vi "周期设置.vi"(11 "定时控制参数输入":T1) -> (3 "定时控制参数输出":T1)   [LabVIEW 2016, in "质控单元.lvlib"]
uses:
  <vilib>/Utility/miscctls.llb/LVPointTypeDef.ctl
panel:
  in  "采配水启用":bool
  in  "模块选择":T2
  in  "确定":bool
  in  "取消":bool
  in  "定时功能启用":bool
  out "选项卡控件":enum32{"定点启动", "间隔启动"}(tab)
  in  "24H周期设置":bool[](xcontrol)
  in  "已经启动次数":dbl
  in  "设定启动次数":dbl
  in  "定时间隔":dbl
  in  "周期设置类型":enum16{"定点启动", "间隔启动"}(ring)
  # "仪器测试类型："
  # "周期设置类型："
  # "请输入定时启动间隔"
  # "min"
  # "次"
  # "次"
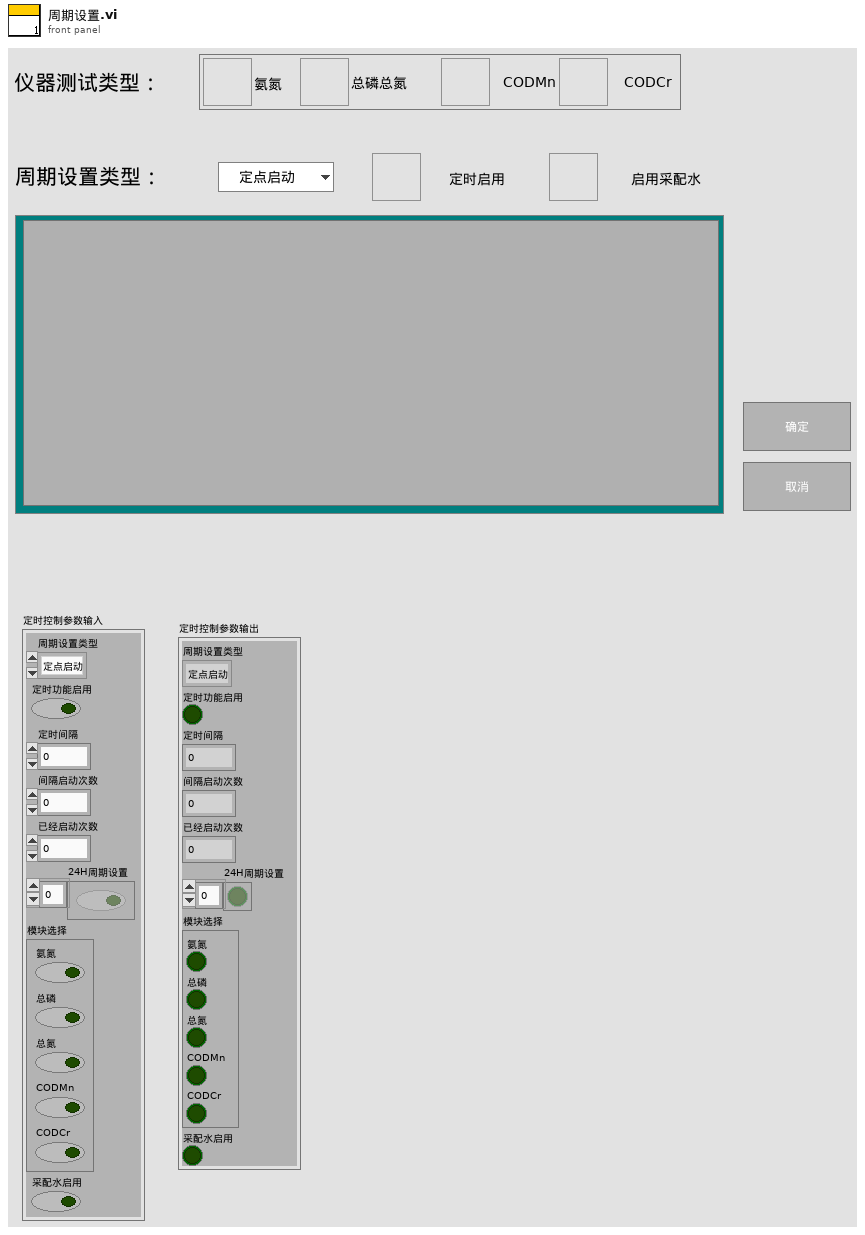
[diagram p1: front panel]
types:
  T1 = cluster{"周期设置类型":enum16{"定点启动", "间隔启动"}, "定时功能启用":bool, "定时间隔":dbl, "间隔启动次数":dbl, "已经启动次数":dbl, "24H周期设置":bool[], "模块选择":cluster{"氨氮":bool, "总磷":bool, "总氮":bool, "CODMn":bool, "CODCr":bool}, "采配水启用":bool}
  T2 = cluster{"氨氮":bool, "总磷":bool, "总氮":bool, "CODMn":bool, "CODCr":bool}
  T3 = typedef "LVPointTypeDef.ctl" = cluster{"Horizontal":i16, "Vertical":i16}
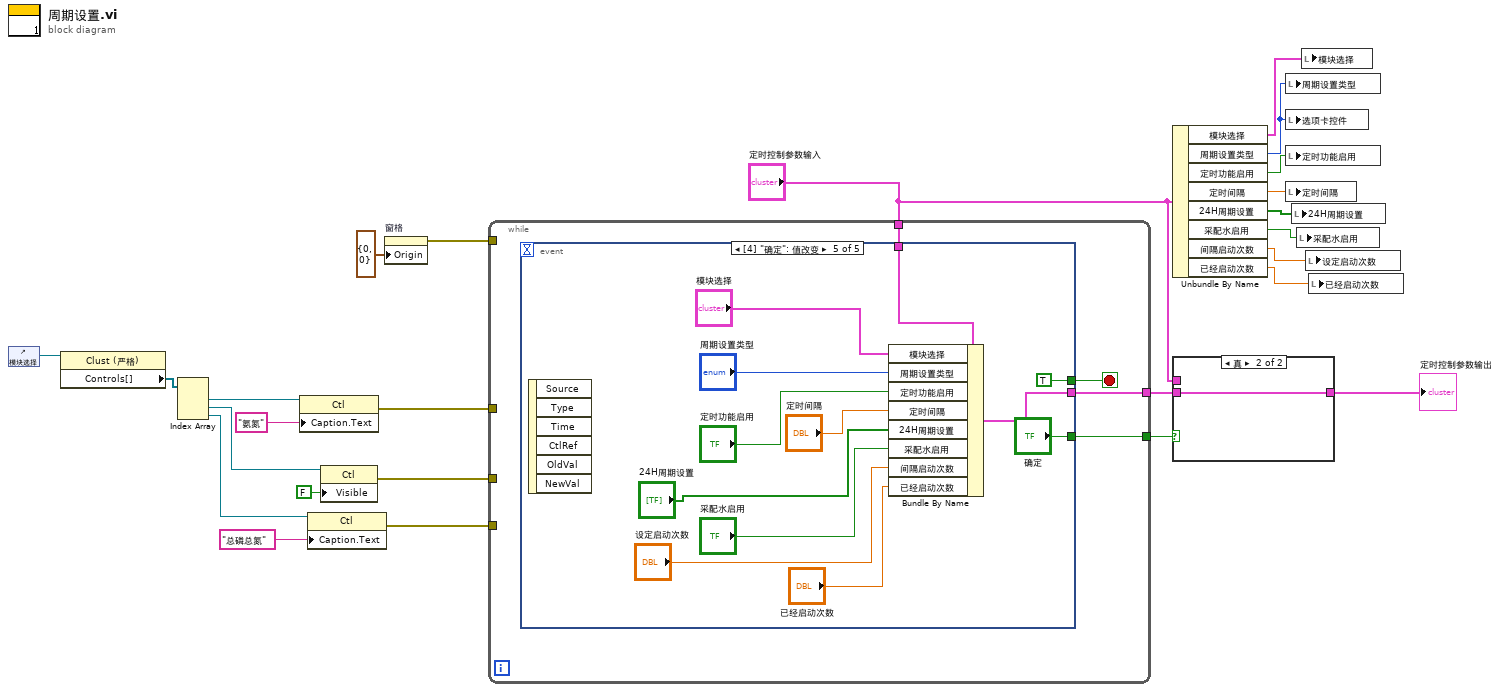
[diagram p0: block diagram]
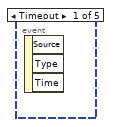
[diagram p3: hidden frame]
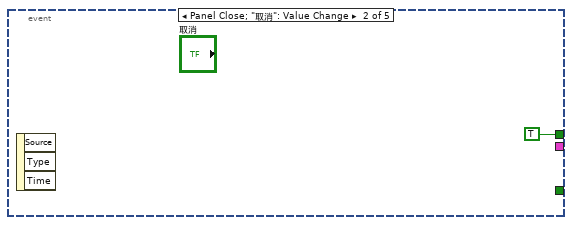
[diagram p4: hidden frame]
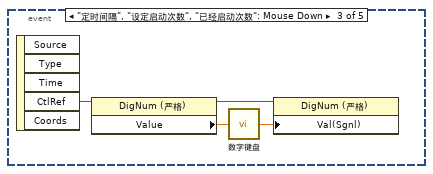
[diagram p5: hidden frame]
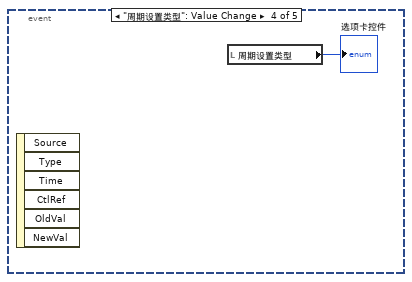
[diagram p6: hidden frame]
diagram:
  n1 = control-ref of="模块选择"() -> (w11:refnum<vi>)
  n2 = property class="Clust (严格)"(reference=w11) -> ("Controls[]"=w9:refnum<vi>[])  [unwired: 1 in, 2 out]
  n3 = Index Array(array=w9) -> (element #1=w10:refnum<vi>, element #2=w7:refnum<vi>, element #3=w2:refnum<vi>)  [unwired: 3 in]
  n4 = property class="Ctl"(reference=w10, "Caption.Text"="氨氮" ("标题.文本")) -> (error out=w5:errorcluster)  [unwired: 1 in, 1 out]
  n5 = property class="Ctl"(reference=w2, "Caption.Text"="总磷总氮" ("标题.文本")) -> (error out=w1:errorcluster)  [unwired: 1 in, 1 out]
  n6 = property class="Ctl"(reference=w7, "Visible"=FALSE ("可见")) -> (error out=w4:errorcluster)  [unwired: 1 in, 1 out]
  n7 = property on="窗格" class="Pane"("Origin"=T3 {"Horizontal"=0, "Vertical"=0} ("原点")) -> (error out=w14:errorcluster)  [unwired: 2 in, 1 out]
  n8 = while {
    tunnel: [w28] -> w20
    tunnel: [w27] -> w21
    tunnel: "定时控制参数输入" -> [w26]
    tunnel: w14 -> [_]
    tunnel: w5 -> [_]
    tunnel: w4 -> [_]
    tunnel: w1 -> [_]
    stop <- w29 stop-if-true
    n9 = event shown="[4] \"确定\": 值改变" {
      selector: _ -> [_ _ _ _ _]
      dyn-events: _ -> [_ _ _ _ _]
      timeout: _ -> [_ _ _ _ _]
      tunnel: [_ TRUE _ _ TRUE] -> w29
      tunnel: [_ _ _ _ w44] -> w28
      tunnel: [_ _ _ _ "确定"] -> w27
      tunnel: w26 -> [_ _ _ _ w39]
      event Timeout {
        n10 = event-data() -> ()  [unwired: 1 in, 3 out]
      }
      event Panel Close; "取消": Value Change {
        n11 = event-data() -> ()  [unwired: 1 in, 3 out]
      }
      event "定时间隔", "设定启动次数", "已经启动次数": Mouse Down {
        n12 = event-data() -> ("CtlRef"=w34:refnum<vi>)  [unwired: 1 in, 4 out]
        n13 = property class="DigNum (严格)"(reference=w34) -> (reference out=w31:refnum<vi>, "Value"=w33:dbl)  [unwired: 1 in, 1 out]
        n14 = call "数字键盘.vi"("OldNumber"=w33) -> ("NewNumber"=w32:sgl)
        n15 = property class="DigNum (严格)"(reference=w31, "Val(Sgnl)"=w32) -> ()  [unwired: 1 in, 2 out]
      }
      event "周期设置类型": Value Change {
        n16 = event-data() -> ()  [unwired: 1 in, 6 out]
        n17 = local read "周期设置类型"() -> (→"选项卡控件":enum16{"定点启动", "间隔启动"})
      }
      event "确定": Value Change {
        n18 = event-data() -> ()  [unwired: 1 in, 6 out]
        n19 = Bundle By Name(cluster=w39, "模块选择"="模块选择", "周期设置类型"="周期设置类型", "定时功能启用"="定时功能启用", "定时间隔"="定时间隔", "24H周期设置"="24H周期设置", "采配水启用"="采配水启用", "间隔启动次数"="设定启动次数", "已经启动次数"="已经启动次数") -> (w44:T1)
      }
    }
  }
  n20 = Unbundle By Name("定时控制参数输入") -> ("模块选择"=w19:T2, "周期设置类型"=w22:enum16{"定点启动", "间隔启动"}, "定时功能启用"=w25:bool, "定时间隔"=w24:dbl, "24H周期设置"=w23:bool[], "采配水启用"=w17:bool, "间隔启动次数"=w13:dbl, "已经启动次数"=w12:dbl)
  n21 = case shown="真" w21 {
    tunnel: w20 -> [_ w49]
    tunnel: [w48 w49] -> w18
    tunnel: "定时控制参数输入" -> [w48 _]
    frame False {
    }
    frame True {
    }
  }
  "定时控制参数输出" <- w18
  n22 = local write "周期设置类型"(w22) -> ()
  n23 = local write "选项卡控件"(w22) -> ()
  n24 = local write "定时功能启用"(w25) -> ()
  n25 = local write "定时间隔"(w24) -> ()
  n26 = local write "24H周期设置"(w23) -> ()
  n27 = local write "采配水启用"(w17) -> ()
  n28 = local write "模块选择"(w19) -> ()
  n29 = local write "设定启动次数"(w13) -> ()
  n30 = local write "已经启动次数"(w12) -> ()
